vi "Launch Nested Models (Mediated).vi"(8 "error in (no error)":errorcluster, 10 "Nested Models":refnum<class "IModel.lvclass">[](array[class]), 11 "IModel in":refnum<class "IModel.lvclass">) -> (0 "error out":errorcluster, 3 "IModel out":refnum<class "IModel.lvclass">)   [LabVIEW 2017, in "IModel.lvlib" / "IModel.lvclass"]
uses:
  IModel.lvclass
  C:/Program Files (x86)/National Instruments/LabVIEW 2017/vi.lib/ActorFramework/Actor/Actor.lvclass
  C:/Git/mva-framework/Source/Framework/IObserver/IObserver/IObserver.lvclass
  IModel.lvclass/IModel.ctl
  IObserver/IObserver/IObserver.lvclass/IObserver.ctl
  IObserver/IObserver/Transfer Observer Resources.vi
  <vilib>/ActorFramework/Actor/Actor.lvclass
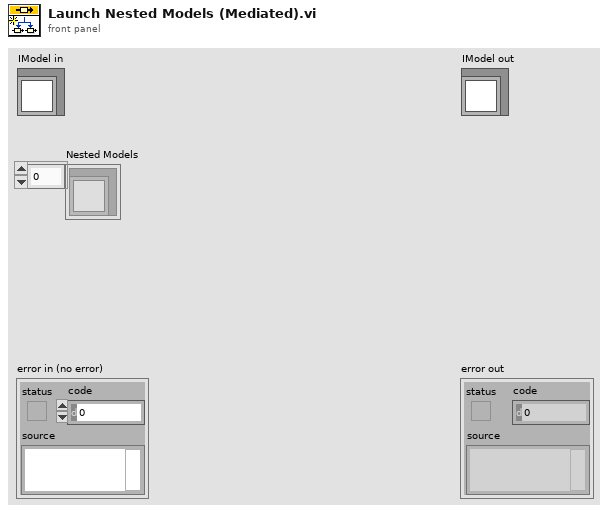
[diagram p1: front panel]
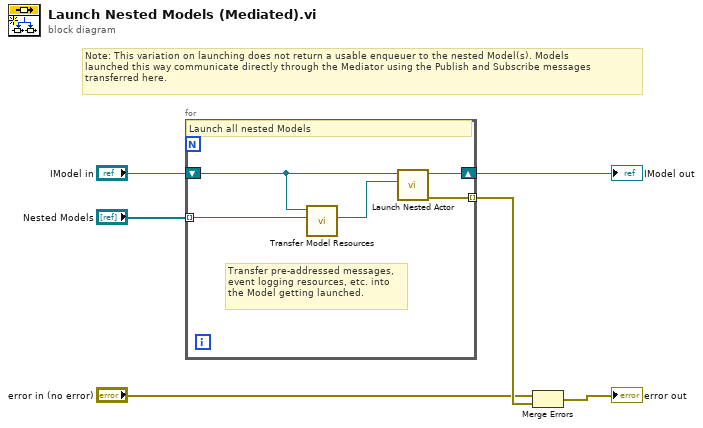
[diagram p0: block diagram]
diagram:
  # "Note: This variation on launching does not return a usable enqueuer to the nested Model(s). Models\nlaunched this way communicate directly through the Mediator using the Publish and Subscribe messages\ntransferred here."
  n1 = for {
    shift-right: [w11] -> w6
    shift-left: "IModel in" -> [w9]
    tunnel: "Nested Models" -> [w8] mode=indexing
    tunnel: [w10] -> w4 mode=indexing
    # "Transfer pre-addressed messages,\nevent logging resources, etc. into\nthe Model getting launched."
    # "Launch all nested Models"
    n2 = call "Transfer Model Resources.vi"("Recipient Model In"=w8, "Running Model"=w9) -> ("Recipient Model Out"=w7:refnum<class "IModel.lvclass">)  [unwired: 9 in]
    n3 = call <vilib>:"Launch Nested Actor.vi"("Nested Actor"=w7, "Caller Actor in"=w9) -> ("error out"=w10:errorcluster, "Caller Actor out"=w11:refnum<class "IModel.lvclass">)  [unwired: 7 in, 1 out]
  }
  "IModel out" <- w6
  n4 = Merge Errors("error in (no error)", w4) -> (→"error out":errorcluster)
